vi "Close.vi"(8 "error in (no error)":errorcluster, 11 "DC Motor Controller in":refnum<class "DC Motor Controller.lvclass">) -> (0 "error out":errorcluster)   [LabVIEW 2019, in "DC Motor Controller.lvclass"]
doc: "Terminates the software connection to the sensor."
uses:
  DC Motor Controller.lvclass
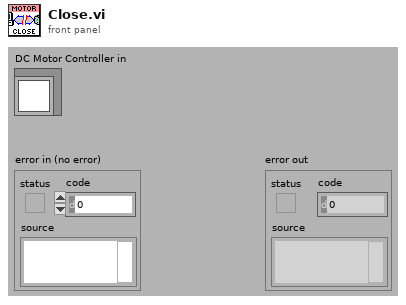
[diagram p1: front panel]
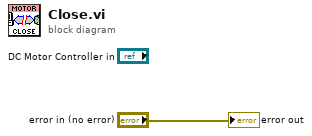
[diagram p0: block diagram]
diagram:
  "error out" <- "error in (no error)"
